vi "HiTechnic SMUX Read.vi"(6 "Offset":u8, 7 "Port":T2 items=["Port 1", "Port 2", "Port 3", "Port 4"], 8 "Parameters":u8[](array[numeric])=[0, 0, 0, 0, 0] format="%x", 9 "Read Length":u8, 10 "MUX Port":u8, 11 "NXT":T1={"error"={"status"=FALSE, "code"=0, "source"=""}, "address"="", "NXT #"=-1, "Show Error"=TRUE, "Connection"=4} {"Connection" items=["USB", "Bluetooth", "USB then Bluetooth", "Last Connection", "Preference"]}) -> (2 "Array":u8[](array[numeric]), 3 "NXT":T1={"error"={"status"=FALSE, "code"=0, "source"=""}, "address"="", "NXT #"=-1, "Show Error"=TRUE, "Connection"=4} {"Connection" items=["USB", "Bluetooth", "USB then Bluetooth", "Last Connection", "Preference"]})   [LabVIEW 2009]
doc: "Reads the Sensor Multiplexer to retrieve data from the selected sensor."
uses:
  <vilib>/NXT/Block Support/NXT_InputPort.ctl
  <vilib>/NXT/Subs/LVHSConnector.ctl
  <vilib>/NXT/Block Support/HWPage.SensorType.ctl
  <vilib>/NXT/Block Support/HWPage.SensorMode.ctl
panel:
  in  "SMUX Initialized":u8[](array[numeric])=[0, 0, 0, 0]
  # "Variables"
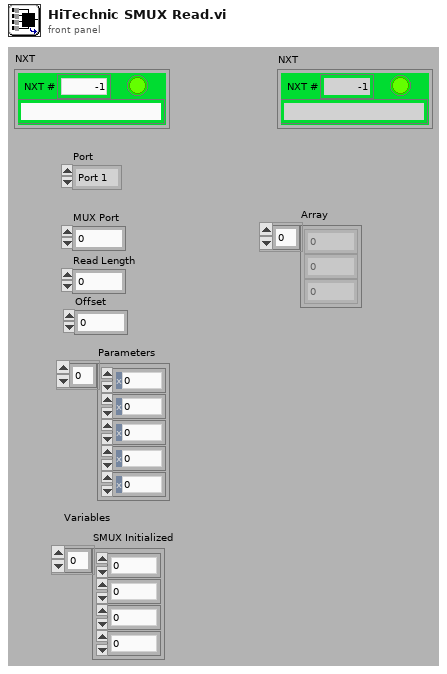
[diagram p1: front panel]
types:
  T1 = typedef "LVHSConnector.ctl" = cluster{"error":errorcluster, "address":string, "NXT #":i32, "Show Error":bool, "Connection":u16}
  T2 = typedef "NXT_InputPort.ctl" = u8
  T3 = typedef "HWPage.SensorType.ctl" = u8
  T4 = typedef "HWPage.SensorMode.ctl" = u8
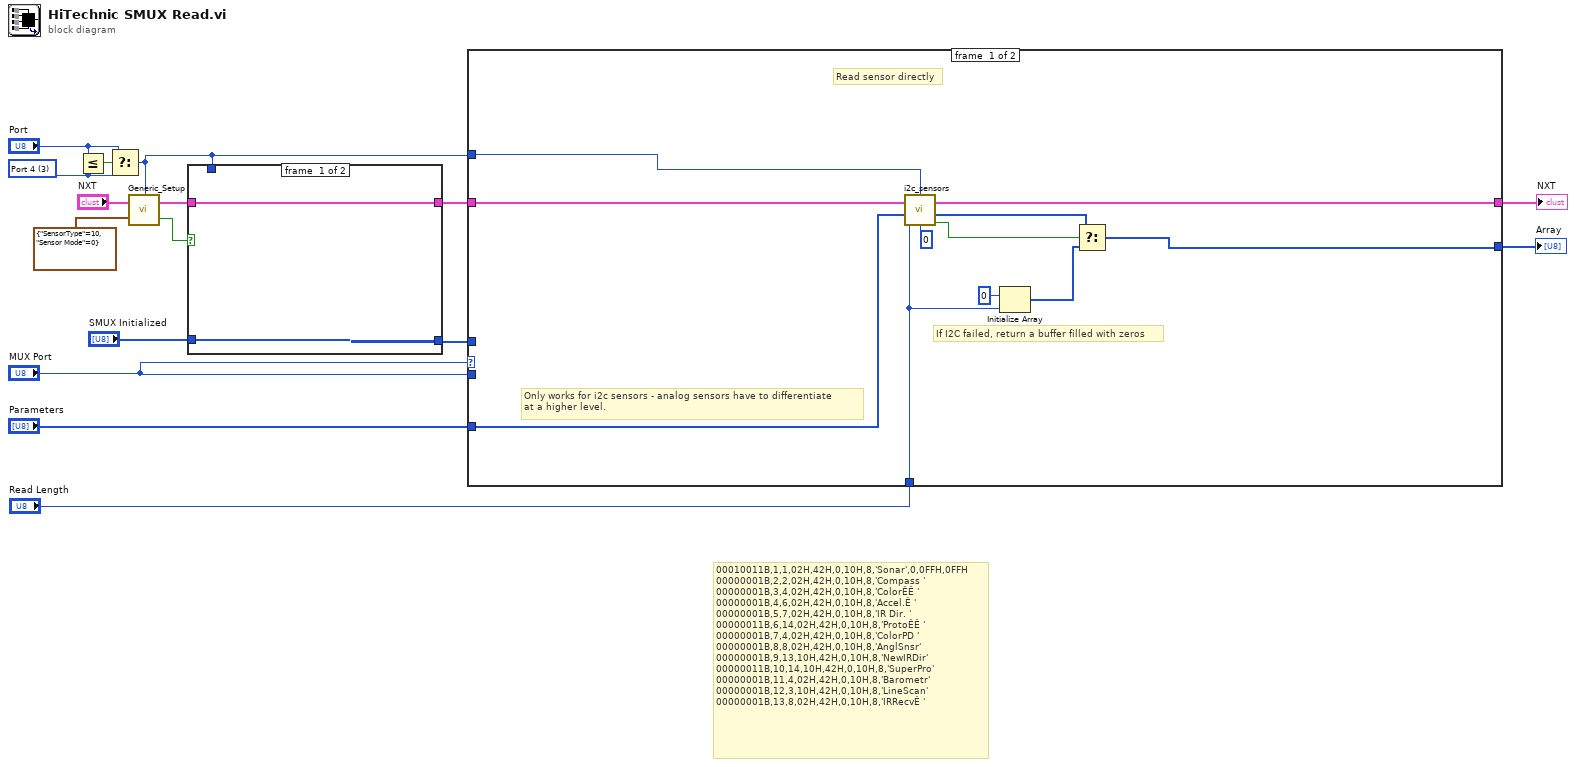
[diagram p0: block diagram]
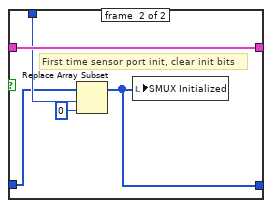
[diagram p2: hidden frame]
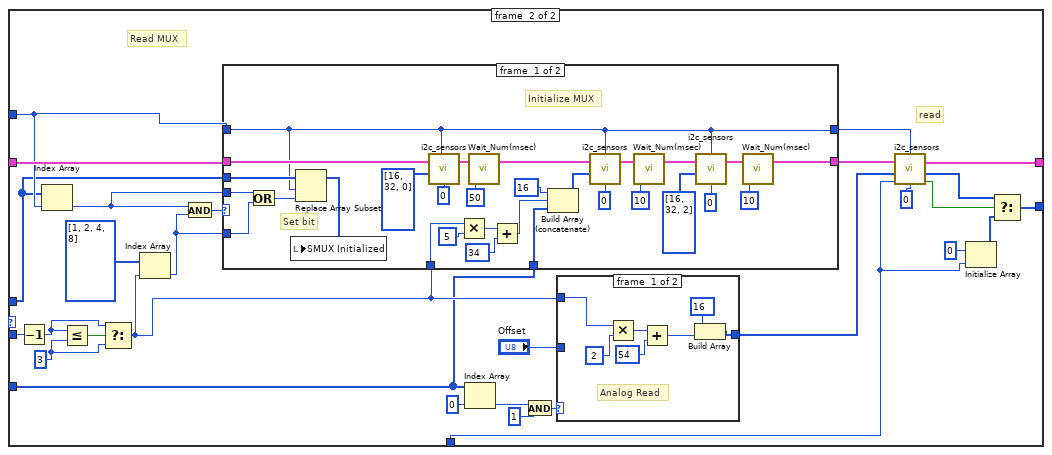
[diagram p3: hidden frame]
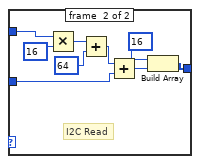
[diagram p4: hidden frame]
diagram:
  w12 = T2 3 items=["Port 1", "Port 2", "Port 3", "Port 4"] ("y")
  # "00010011B,1,1,02H,42H,0,10H,8,'Sonar',0,0FFH,0FFH\n00000001B,2,2,02H,42H,0,10H,8,'Compass '\n00000001B,3,4,02H,42H,0,10H,8,'ColorÊÊ '\n00000001B,4,6,02H,42H,0,10H,8,'Accel.Ê '\n00000001B,5,7,02H,42H,0,10H,8,'IR Dir. '\n00000011B,6,14,02H,42H,0,10H,8,'ProtoÊÊ '\n00000001B,7,4,02H,42H,0,10H,8,'ColorPD '\n00000001B,8,8,02H,42H,0,10H,8,'AnglSnsr'\n00000001B,9,13,10H,42H,0,10H,8,'NewIRDir'\n00000011B,10,14,10H,42H,0,10H,8,'SuperPro'\n00000001B,11,4,02H,42H,0,10H,8,'Barometr'\n00000001B,12,3,10H,42H,0,10H,8,'LineScan'\n00000001B,13,8,02H,42H,0,10H,8,'IRRecvÊ '"
  n1 = Less Or Equal?(x="Port", y=w12) -> (x <= y?=w13:bool)
  n2 = Select(t="Port", s=w13, f=w12) -> (s? t:f=w7:T2)
  n3 = call <vilib>:"Generic_Setup.vi"("Sensor Setup"=cluster{"SensorType":T3, "Sensor Mode":T4} {"SensorType"=10, "Sensor Mode"=0}, "NXT"="NXT", "Port"=w7) -> ("Changed?"=w4:bool, "NXT"=w3:T1)
  n4 = case shown="True" w4 {
    tunnel: [w17 w23] -> w1
    tunnel: w3 -> [w17 w23]
    tunnel: w7 -> [_ w22]
    tunnel: "SMUX Initialized" -> [w18 w20]
    tunnel: [w18 w19] -> w5
    frame #0 {
    }
    frame #1 {
      # "First time sensor port init, clear init bits"
      n5 = Replace Array Subset(array=w20, new element=u8 0 ("new element/subarray"), index=w22) -> (w19:u8[])
      n6 = local write "SMUX Initialized"(w19) -> ()
    }
  }
  n7 = case shown="Default" "MUX Port" {
    tunnel: [w24 w47] -> w16
    tunnel: w7 -> [w25 w46]
    tunnel: "Parameters" -> [w34 w42]
    tunnel: "MUX Port" -> [_ w63]
    tunnel: w1 -> [w29 w50]
    tunnel: [w33 w62] -> w2
    tunnel: "Read Length" -> [w28 w37]
    tunnel: w5 -> [_ w41]
    frame #0 {
      # "If I2C failed, return a buffer filled with zeros"
      # "Only works for i2c sensors - analog sensors have to differentiate \nat a higher level."
      # "Read sensor directly"
      n8 = call <vilib>:"i2c_sensors.vi"("Return Length"=w28, "Bytes to Write"=w34, "Wait (msec)"=u32 0, "NXT"=w29, "Port"=w25) -> ("Success?"=w30:bool, "Bytes read"=w31:u8[], "NXT"=w33:T1)
      n9 = Initialize Array(u8 0 ("element"), w28) -> (w26:u8[])
      n10 = Select(t=w31, s=w30, f=w26) -> (s? t:f=w24:u8[])
    }
    frame #1 {
      w59 = u8 3 ("y")
      # "read"
      # "Read MUX"
      n11 = Decrement(x=w63) -> (x-1=w60:u8)
      n12 = Index Array(array=w41, index=w46) -> (element=w40:u8)
      n13 = Less Or Equal?(x=w60, y=w59) -> (x <= y?=w61:bool)
      n14 = Select(t=w60, s=w61, f=w59) -> (s? t:f=w44:u8)
      n15 = Index Array(array=u8[] [1, 2, 4, 8], index=w44) -> (element=w39:u8)
      n16 = And(x=w40, y=w39) -> (x .and. y?=w43:u8)
      n17 = case shown="0" w43 {
        tunnel: w50 -> [w86 w109]
        tunnel: w46 -> [w81 w110]
        tunnel: w42 -> [w98 _]
        tunnel: [w87 w109] -> w36
        tunnel: [w81 w110] -> w51
        tunnel: w44 -> [w100 _]
        tunnel: w41 -> [w82 _]
        tunnel: w40 -> [w85 _]
        tunnel: w39 -> [w84 _]
        frame #0 {
          # "Set bit"
          # "Initialize MUX"
          n18 = Or(x=w85, y=w84) -> (x .or. y?=w83:u8)
          n19 = Replace Array Subset(array=w82, new element=w83, index=w81) -> (w80:u8[])
          n20 = local write "SMUX Initialized"(w80) -> ()
          n21 = call <vilib>:"i2c_sensors.vi"("Bytes to Write"=u8[] [16, 32, 0], "Wait (msec)"=u32 0, "NXT"=w86, "Port"=w81) -> ("NXT"=w94:T1)  [unwired: 1 in, 2 out]
          n22 = Multiply(x=w100, y=u8 5 ("ReturnLength")) -> (x*y=w102:u8)
          n23 = call <vilib>:"Wait_Num(msec).vi"("Time (msec)"=u32 50, "NXT"=w94) -> ("NXT"=w93:T1)  [unwired: 2 in]
          n24 = Add(x=w102, y=u8 34) -> (x+y=w99:u8)
          n25 = Build Array (concatenate)(u8 16, w99, w98) -> (w97:u8[])
          n26 = call <vilib>:"i2c_sensors.vi"("Bytes to Write"=w97, "Wait (msec)"=u32 0, "NXT"=w93, "Port"=w81) -> ("NXT"=w91:T1)  [unwired: 1 in, 2 out]
          n27 = call <vilib>:"Wait_Num(msec).vi"("Time (msec)"=u32 10, "NXT"=w91) -> ("NXT"=w90:T1)  [unwired: 2 in]
          n28 = call <vilib>:"i2c_sensors.vi"("Bytes to Write"=u8[] [16, 32, 2], "Wait (msec)"=u32 0, "NXT"=w90, "Port"=w81) -> ("NXT"=w88:T1)  [unwired: 1 in, 2 out]
          n29 = call <vilib>:"Wait_Num(msec).vi"("Time (msec)"=u32 10, "NXT"=w88) -> ("NXT"=w87:T1)  [unwired: 2 in]
        }
        frame #1 {
          # "Already initialized"
        }
      }
      n30 = Index Array(array=w42, index=0) -> (element=w56:u8)
      n31 = And(x=w56, y=u8 1) -> (x .and. y?=w57:u8)
      n32 = case shown="1" w57 {
        tunnel: w44 -> [w65 w75]
        tunnel: "Offset" -> [_ w73]
        tunnel: [w64 w71] -> w54
        frame #0 {
          # "Analog Read"
          n33 = Multiply(x=w65, y=u8 2 ("ReturnLength")) -> (x*y=w67:u8)
          n34 = Add(x=w67, y=u8 54) -> (x+y=w70:u8)
          n35 = Build Array(u8 16, w70) -> (w64:u8[])
        }
        frame #1 {
          # "I2C Read"
          n36 = Multiply(x=w75, y=u8 16 ("ReturnLength")) -> (x*y=w78:u8)
          n37 = Add(x=w78, y=u8 64) -> (x+y=w74:u8)
          n38 = Add(x=w74, y=w73) -> (x+y=w72:u8)
          n39 = Build Array(u8 16, w72) -> (w71:u8[])
        }
      }
      n40 = call <vilib>:"i2c_sensors.vi"("Return Length"=w37, "Bytes to Write"=w54, "Wait (msec)"=u32 0, "NXT"=w36, "Port"=w51) -> ("Success?"=w35:bool, "Bytes read"=w38:u8[], "NXT"=w62:T1)
      n41 = Initialize Array(u8 0 ("element"), w37) -> (w48:u8[])
      n42 = Select(t=w38, s=w35, f=w48) -> (s? t:f=w47:u8[])
    }
  }
  "Array" <- w16
  "NXT" <- w2
